vi "WFComposeD.vi"(7 "Inverted":bool, 8 "error in (no error)":errorcluster, 10 "WFRepetitions":T1={"Del (s)"=0.0, "Int (s)"=0.0, "N"=1} {"Int (s)" min=0.0 format="%#_4g"; "Del (s)" min=0.0 format="%#_4f"}, 11 "Waveform In":digitalwaveform(waveform)={"t0"=timestamp(0 s since 1904-01-01), "dt"=1.0, "Y"={"transitions"=[], "data"=[[0, 0, 0, 1], [0, 1, 0, 0]]}}) -> (0 "error out":errorcluster, 3 "Waveform Out":digitalwaveform(waveform)={"t0"=timestamp(0 s since 1904-01-01), "dt"=1.0, "Y"={"transitions"=[], "data"=[[0, 0, 0, 1], [0, 1, 0, 0]]}})   [LabVIEW 2013]
uses:
  WFRepetitions.ctl
  WFComposeCanD.vi
  WFGetDtFsD.vi
  <vilib>/Waveform/DWDTOps.llb/DWDT Digital Size.vi
  <vilib>/Waveform/DWDTOps.llb/DWDT Boolean Array to Digital.vi
  WFAppend2D.vi
  <vilib>/Waveform/DWDTOps.llb/DWDT Invert Digital.vi
panel:
  out "Digital Waveform Graph":digitalwaveform(graph)
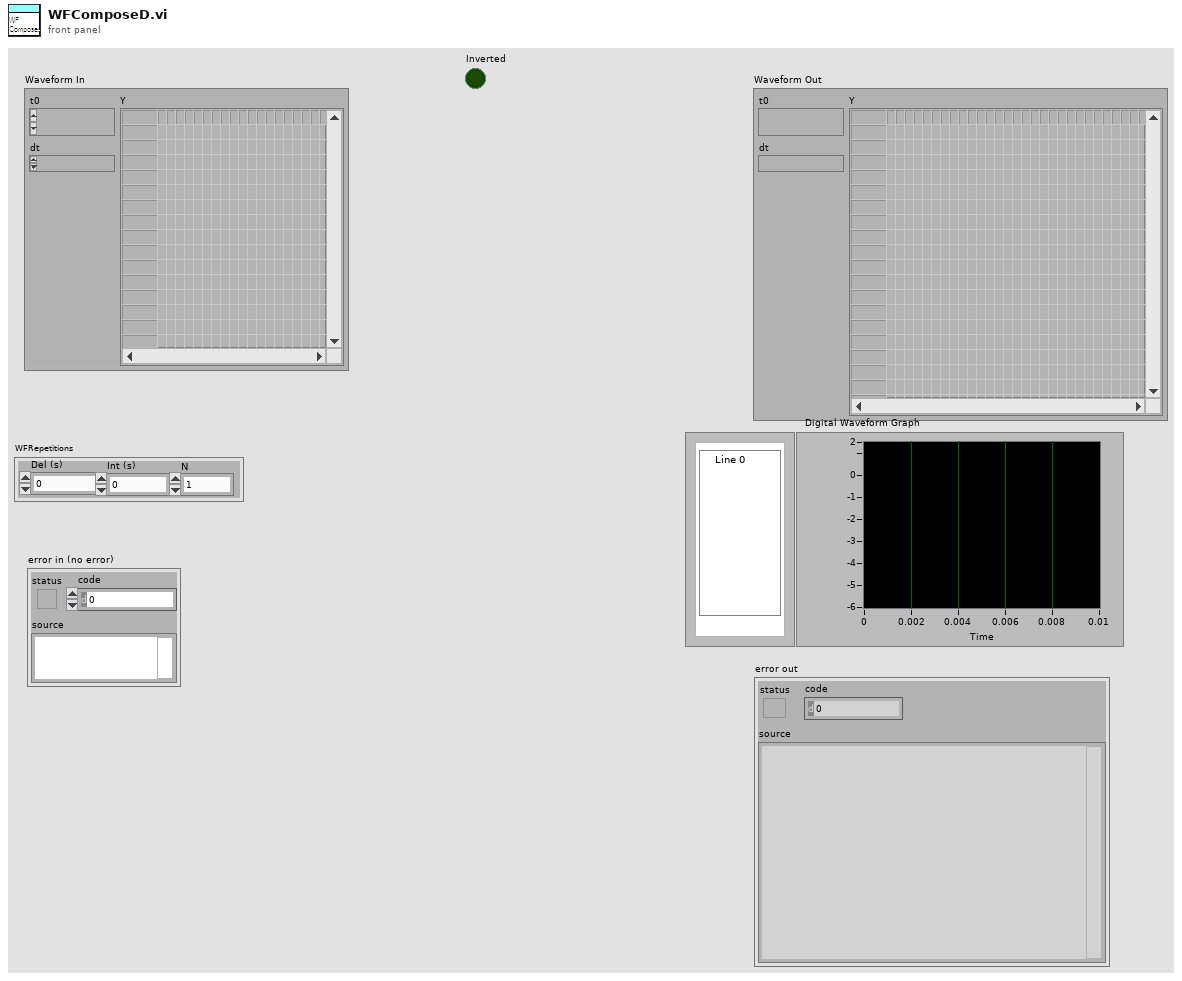
[diagram p1: front panel]
types:
  T1 = typedef "WFRepetitions.ctl" = cluster{"Del (s)":dbl, "Int (s)":dbl, "N":i32}
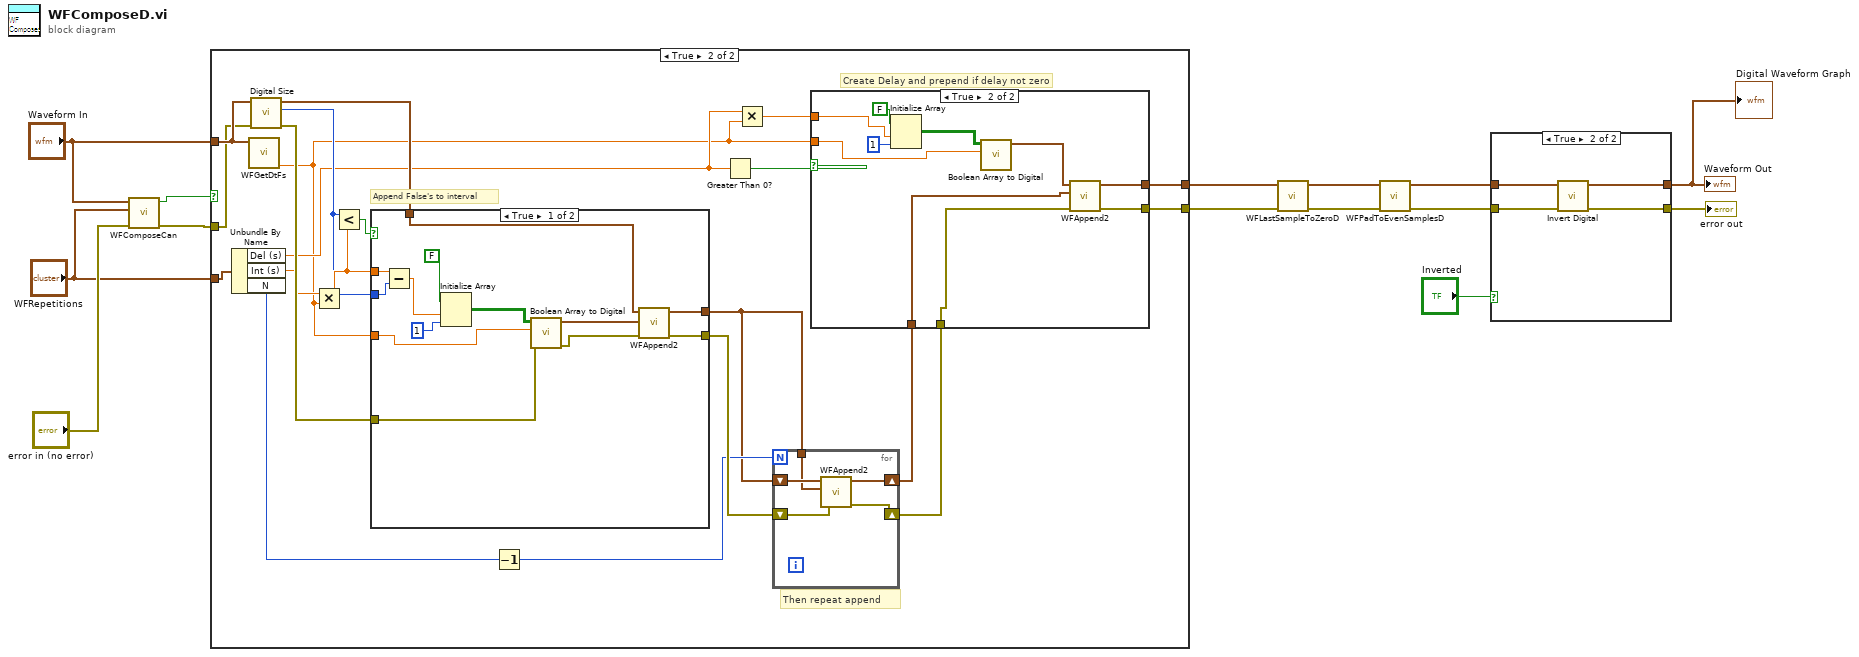
[diagram p0: block diagram]
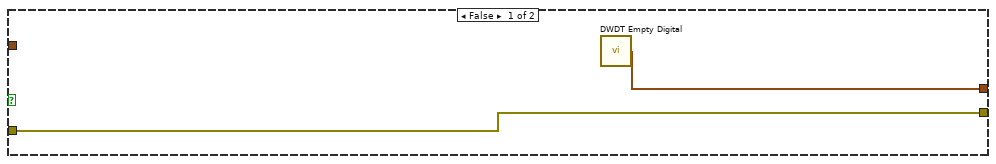
[diagram p3: hidden frame]
diagram:
  n1 = call-poly "WFComposeCan.vi"("error in (no error)"="error in (no error)", "Cluster"="WFRepetitions", "Waveform In"="Waveform In") -> ("error out"=w12:errorcluster, "ComposeCan"=w14:bool)  [unwired: 7 in]
  n2 = case shown="True" w14 {
    tunnel: [w15 w25] -> w4
    tunnel: w12 -> [w16 w31]
    tunnel: [w16 w23] -> w2
    tunnel: "Waveform In" -> [_ w34]
    tunnel: "WFRepetitions" -> [_ w35]
    frame False {
      n3 = call <vilib>:"DWDT Empty Digital.vi"() -> ("digital waveform out"=w15:digitalwaveform)  [unwired: 5 in]
    }
    frame True {
      # "Then repeat append"
      # "Create Delay and prepend if delay not zero"
      # "Append False's to interval"
      n4 = Unbundle By Name(w35) -> ("Del (s)"=w19:dbl, "Int (s)"=w22:dbl, "N"=w29:i32)
      n5 = call-poly "WFGetDtFs.vi"("Waveform"=w34) -> ("Fs (Hz)"=w17:dbl)  [unwired: 9 in, 1 out]
      n6 = call-poly <vilib>:"Digital Size.vi"("error in (no error)"=w31, "digital waveform in"=w34) -> ("error out"=w30:errorcluster, "number of samples"=w20:i32, "digital waveform out"=w32:digitalwaveform)  [unwired: 6 in, 1 out]
      n7 = Multiply(x=w22, y=w17) -> (x*y=w21:dbl)
      n8 = Less?(x=w20, y=w21) -> (x < y?=w33:bool)
      n9 = case shown="True" w33 {
        tunnel: [w53 w57] -> w36
        tunnel: [w52 w56] -> w27
        tunnel: w32 -> [w46 w56]
        tunnel: w21 -> [w45 _]
        tunnel: w30 -> [w49 w57]
        tunnel: w20 -> [w44 _]
        tunnel: w17 -> [w43 _]
        frame True {
          n10 = Subtract(x=w45, y=w44) -> (x-y=w54:dbl)
          n11 = Initialize Array(FALSE, w54, 1 ("dimension size")) -> (w50:bool[][])
          n12 = call-poly <vilib>:"Boolean Array to Digital.vi"("error in (no error)"=w49, "sample rate"=w43, "boolean array"=w50) -> ("error out"=w48:errorcluster, "digital waveform"=w47:digitalwaveform)  [unwired: 7 in]
          n13 = call-poly "WFAppend2.vi"("error in (no error)"=w48, "Waveform In 2"=w47, "Waveform In"=w46) -> ("error out"=w53:errorcluster, "Waveform Out"=w52:digitalwaveform)  [unwired: 3 in]
        }
        frame False {
        }
      }
      n14 = Decrement(x=w29) -> (x-1=w28:i32)
      n15 = Greater Than 0?(x=w19) -> (x > 0?=w37:bool)
      n16 = Multiply(x=w19, y=w17) -> (x*y=w18:dbl)
      n17 = for {
        N: w28 -> [_]
        shift-right: [w41] -> w26
        shift-left: w27 -> [w42]
        shift-right: [w39] -> w24
        shift-left: w36 -> [w40]
        tunnel: w27 -> [w38]
        n18 = call-poly "WFAppend2.vi"("error in (no error)"=w40, "Waveform In 2"=w38, "Waveform In"=w42) -> ("error out"=w39:errorcluster, "Waveform Out"=w41:digitalwaveform)  [unwired: 3 in]
      }
      n19 = case shown="True" w37 {
        tunnel: w17 -> [_ w64]
        tunnel: w26 -> [w59 w62]
        tunnel: [w59 w61] -> w25
        tunnel: w24 -> [w58 w69]
        tunnel: [w58 w68] -> w23
        tunnel: w18 -> [_ w60]
        frame False {
        }
        frame True {
          n20 = Initialize Array(FALSE, w60, 1 ("dimension size")) -> (w65:bool[][])
          n21 = call-poly <vilib>:"Boolean Array to Digital.vi"("sample rate"=w64, "boolean array"=w65) -> ("digital waveform"=w63:digitalwaveform)  [unwired: 8 in, 1 out]
          n22 = call-poly "WFAppend2.vi"("error in (no error)"=w69, "Waveform In 2"=w62, "Waveform In"=w63) -> ("error out"=w68:errorcluster, "Waveform Out"=w61:digitalwaveform)  [unwired: 3 in]
        }
      }
    }
  }
  n23 = call "WFLastSampleToZeroD.vi"("error in (no error)"=w2, "Waveform In"=w4) -> ("error out"=w1:errorcluster, "Waveform Out"=w3:digitalwaveform)  [unwired: 4 in]
  n24 = call "WFPadToEvenSamplesD.vi"("error in (no error)"=w1, "Waveform In"=w3) -> ("error out"=w5:errorcluster, "Waveform Out"=w6:digitalwaveform)  [unwired: 4 in]
  n25 = case shown="True" "Inverted" {
    tunnel: w6 -> [w71 w75]
    tunnel: [w71 w74] -> w7
    tunnel: w5 -> [w70 w73]
    tunnel: [w70 w72] -> w8
    frame False {
    }
    frame True {
      n26 = call-poly <vilib>:"Invert Digital.vi"("error in (no error)"=w73, "digital waveform"=w75) -> ("error out"=w72:errorcluster, "inverted waveform"=w74:digitalwaveform)  [unwired: 8 in]
    }
  }
  "error out" <- w8
  "Waveform Out" <- w7
  "Digital Waveform Graph" <- w7
